vi "MagX Sort Info.vi"(8 "error in":errorcluster, 11 "Data in":T1[](array[typedef])) -> (0 "error out":errorcluster, 3 "Data out":T1[](array[typedef]))   [LabVIEW 2021]
uses:
  Experiment info.ctl
  4e327397-afd7-435d-a89f-99371f95702d.vi
  <vilib>/Comparison/Less/Less Functor/Less Functor.lvclass
panel:
  out "Array":timestamp[](array[timestamp])
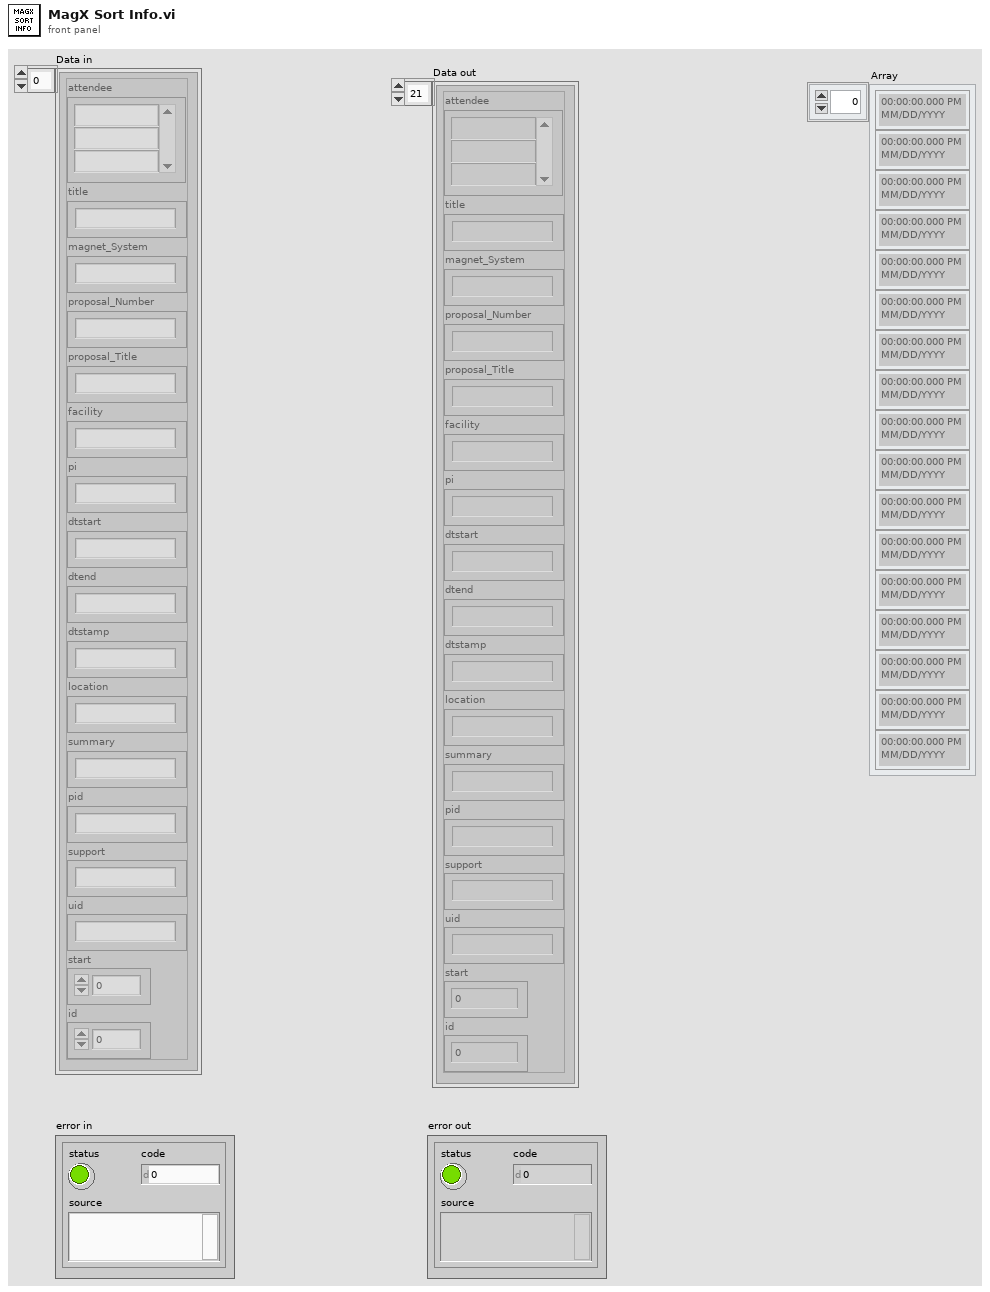
[diagram p1: front panel]
types:
  T1 = typedef "Experiment info.ctl" = cluster{"attendee":string[], "title":string, "magnet_System":string, "proposal_Number":string, "proposal_Title":string, "facility":string, "pi":string, "dtstart":string, "dtend":string, "dtstamp":string, "location":string, "summary":string, "pid":string, "support":string, "uid":string, "start":u64, "id":u64}
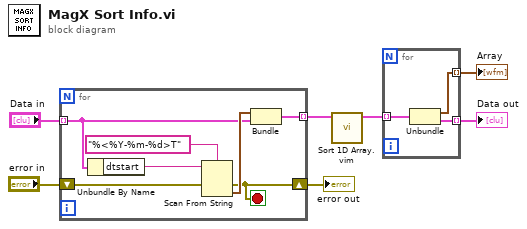
[diagram p0: block diagram]
diagram:
  n1 = for {
    tunnel: "Data in" -> [w11] mode=indexing
    tunnel: [w10] -> w6 mode=indexing
    shift-right: [w8] -> w1
    shift-left: "error in" -> [w9]
    stop <- w8 stop-if-true
    n2 = Unbundle By Name(w11) -> ("dtstart"=w14:string)
    n3 = Scan From String(format string="%<%Y-%m-%d>T", input string=w14, error in=w9) -> (error out=w8:errorcluster, output 1=w12:timestamp)  [unwired: 2 in, 2 out]
    n4 = Bundle(w12, "Experiment info"=w11) -> (w10:cluster{timestamp, "Experiment info":T1})  [unwired: 1 in]
  }
  "error out" <- w1
  n5 = call "Sort 1D Array.vim"("unsorted array"=w6) -> ("sorted array"=w5:cluster{timestamp, "Experiment info":T1}[])  [unwired: 10 in]
  n6 = for {
    tunnel: w5 -> [w17] mode=indexing
    tunnel: [w16] -> w4 mode=indexing
    tunnel: [w15] -> w3 mode=indexing
    n7 = Unbundle(w17) -> (w15:timestamp, "Experiment info"=w16:T1)
  }
  "Data out" <- w4
  "Array" <- w3
